vi "BRig_dataRT_stats__BUR_target.vi"() -> (2 "output_BUR_target":i32)   [LabVIEW 2014]
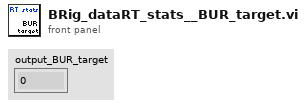
[diagram p1: front panel]
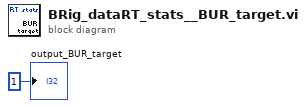
[diagram p0: block diagram]
diagram:
  "output_BUR_target" <- 1 ("output_iBlock")
